vi "Read VISA resource name.vi"(8 "error in (no error)":errorcluster, 11 "INL Valve Controller in":refnum<class "INL Valve Controller.lvclass">) -> (0 "error out":errorcluster, 2 "VISA resource name":refnum<visa-resource-name>, 3 "INL Valve Controller out":refnum<class "INL Valve Controller.lvclass">)   [LabVIEW 2011, in "INL Valve Controller.lvclass"]
uses:
  INL Valve Controller.lvclass
  INL Valve Controller.lvclass/INL Valve Controller.ctl
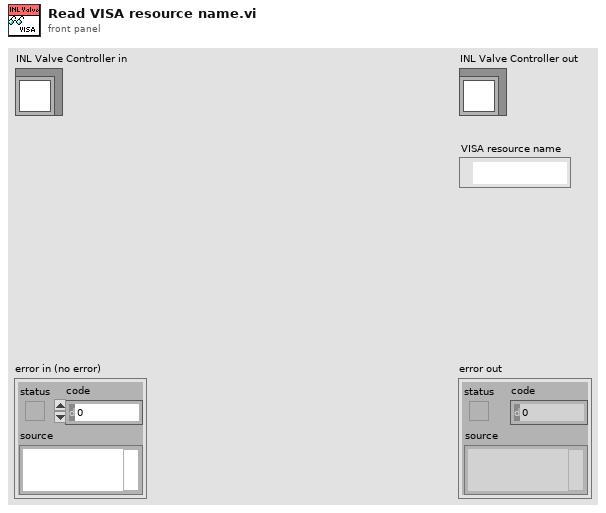
[diagram p1: front panel]
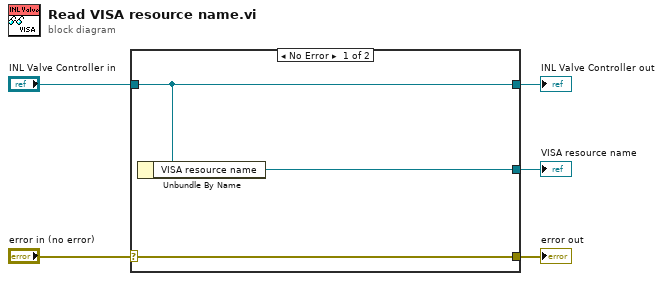
[diagram p0: block diagram]
diagram:
  n1 = case shown="No Error" "error in (no error)" {
    selector: "error in (no error)" -> [w8 w9]
    tunnel: [w8 w9] -> w4
    tunnel: [w7 w10] -> w2
    tunnel: "INL Valve Controller in" -> [w7 w10]
    tunnel: [w6 _] -> w1
    frame No Error {
      n2 = Unbundle By Name(w7) -> ("VISA resource name"=w6:refnum<visa-resource-name>)
    }
    frame Error {
    }
  }
  "error out" <- w4
  "INL Valve Controller out" <- w2
  "VISA resource name" <- w1
